vi "Sub.vi"(8 "error in (no error)":errorcluster caption="错误输入（无错误）", 10 "Point 输入":refnum<class "Point.lvclass"> caption="DNL_LabVIEW Object in", 11 "Point 输入":refnum<class "Point.lvclass"> caption="DNL_LabVIEW Object in") -> (0 "error out":errorcluster caption="错误输出", 3 "Point 输出":refnum<class "Point.lvclass"> caption="DNL_LabVIEW Object out")   [LabVIEW 2011, in "Point.lvclass"]
uses:
  Point.lvclass
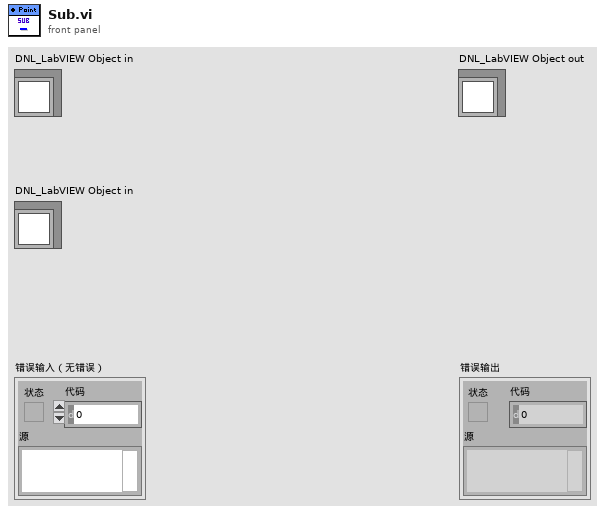
[diagram p1: front panel]
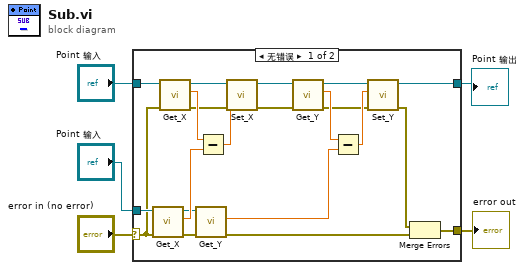
[diagram p0: block diagram]
diagram:
  n1 = case shown="无错误" "error in (no error)" {
    selector: "error in (no error)" -> [w20 w28]
    tunnel: [w7 w28] -> w4
    tunnel: [w10 w27] -> w3
    tunnel: "Point 输入" -> [w26 w27]
    tunnel: "Point 输入" -> [w25 _]
    frame No Error {
      n2 = call "Get_X.vi"("error in (no error)"=w20, "Point输入"=w25) -> ("error out"=w18:errorcluster, "X"=w23:dbl, "Point输出"=w19:refnum<class "Point.lvclass">)  [unwired: 7 in]
      n3 = call "Get_X.vi"("error in (no error)"=w20, "Point输入"=w26) -> ("error out"=w6:errorcluster, "X"=w24:dbl, "Point输出"=w22:refnum<class "Point.lvclass">)  [unwired: 7 in]
      n4 = call "Get_Y.vi"("error in (no error)"=w18, "Point输入"=w19) -> ("error out"=w8:errorcluster, "Y"=w14:dbl)  [unwired: 7 in, 1 out]
      n5 = Subtract(x=w24, y=w23) -> (x-y=w21:dbl)
      n6 = call "Set_X.vi"("error in (no error)"=w6, "X"=w21, "Point输入"=w22) -> ("error out"=w16:errorcluster, "Point输出"=w17:refnum<class "Point.lvclass">)  [unwired: 7 in]
      n7 = call "Get_Y.vi"("error in (no error)"=w16, "Point输入"=w17) -> ("error out"=w11:errorcluster, "Y"=w15:dbl, "Point输出"=w13:refnum<class "Point.lvclass">)  [unwired: 7 in]
      n8 = Subtract(x=w15, y=w14) -> (x-y=w12:dbl)
      n9 = call "Set_Y.vi"("error in (no error)"=w11, "Y"=w12, "Point输入"=w13) -> ("error out"=w9:errorcluster, "Point输出"=w10:refnum<class "Point.lvclass">)  [unwired: 7 in]
      n10 = Merge Errors(w9, w8) -> (w7:errorcluster)
    }
    frame Error {
    }
  }
  "error out" <- w4
  "Point 输出" <- w3
